vi "Destroy Request Events.vi"(8 "error in":errorcluster) -> (0 "error out":errorcluster)   [LabVIEW 2024, in "Singleton Subpanel.lvlib"]
doc: "Destroy the requests user events, even if there is an incoming error.\n\n<b>NOTE</b>: The contents of this VI are automatically generated and modified by the <b>Tools > DQMH Consortium > DQMH</b> utilities. Consider using those utilities instead of making your own modifications to this VI.\n_____\nBased on DQMH Dev Tools: Project Template 7.1.0.1499."
uses:
  Singleton Subpanel.lvlib
panel:
  # "NOTE: The contents of this VI are automatically generated and modified by the Tools > DQMH Consortium > DQMH utilities. Consider using those utilities instead of making your own modifications to this VI."
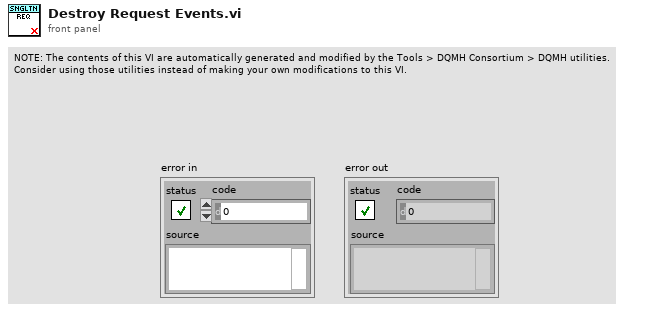
[diagram p1: front panel]
types:
  T1 = typedef "Singleton Subpanel.lvlib/Request Events--cluster.ctl" = cluster{"Stop Module":refnum<user-event>, "Show Panel":refnum<user-event>, "Hide Panel":refnum<user-event>, "Get Module Execution Status":refnum<user-event>, "Show Diagram":refnum<user-event>, "Draw FP in SubPanel":refnum<user-event>, "Remove from SubPanel":refnum<user-event>}
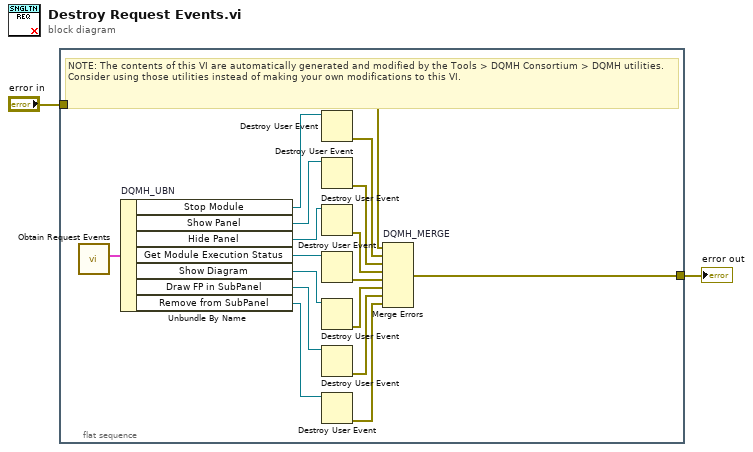
[diagram p0: block diagram]
diagram:
  n1 = flat-sequence {
    tunnel: [w18] -> w2
    tunnel: "error in" -> [w11]
    frame #0 {
      # "NOTE: The contents of this VI are automatically generated and modified by the Tools > DQMH Consortium > DQMH utilities. Consider using those utilities instead of making your own modifications to this VI."
      n2 = call "Obtain Request Events.vi"() -> ("Singleton Subpanel Request Events"=w17:T1)  [unwired: 10 in, 1 out]
      n3 = Unbundle By Name "DQMH_UBN"(w17) -> ("Stop Module"=w16:refnum<user-event>, "Show Panel"=w13:refnum<user-event>, "Hide Panel"=w12:refnum<user-event>, "Get Module Execution Status"=w9:refnum<user-event>, "Show Diagram"=w7:refnum<user-event>, "Draw FP in SubPanel"=w5:refnum<user-event>, "Remove from SubPanel"=w3:refnum<user-event>)
      n4 = Destroy User Event(user event=w16) -> (error out=w19:errorcluster)  [unwired: 1 in]
      n5 = Destroy User Event(user event=w13) -> (error out=w15:errorcluster)  [unwired: 1 in]
      n6 = Destroy User Event(user event=w12) -> (error out=w14:errorcluster)  [unwired: 1 in]
      n7 = Destroy User Event(user event=w9) -> (error out=w10:errorcluster)  [unwired: 1 in]
      n8 = Destroy User Event(user event=w7) -> (error out=w8:errorcluster)  [unwired: 1 in]
      n9 = Destroy User Event(user event=w5) -> (error out=w6:errorcluster)  [unwired: 1 in]
      n10 = Destroy User Event(user event=w3) -> (error out=w4:errorcluster)  [unwired: 1 in]
      n11 = Merge Errors "DQMH_MERGE"(w11, w19, w15, w14, w10, w8, w6, w4) -> (w18:errorcluster)
    }
  }
  "error out" <- w2
